vi "Fancy Dialog Box (LVOOP).vi"() -> ()   [LabVIEW 2012]
doc: "This example shows how to use the UI Tools Dialog classes to create fancy dialog boxes with background blackening."
uses:
  _Commands_Example.ctl
  Dialog/Dialog/Dialog/Dialog.lvclass
  Dialog/ListSelection/Selection Mode.ctl
  Dialog/MessageBox/pictures/pictures.ctl
  Fading/_Fade In(I32).vi
  Fading/_Fade Out(I32).vi
  Dialog/MessageBox/MessageBox.lvclass
  Dialog/Msg_Error/Msg_Error.lvclass
  Dialog/ListSelection/ListSelection.lvclass
panel:
  in  "Error\nDialog":bool caption="Press this button to simulate a dialog box call."
  in  "Alarm\nDialog":bool caption="Press this button to simulate a dialog box call."
  in  "Selection\nList":bool caption="Press this button to simulate a dialog box call."
  in  "One-button\nDialog":bool caption="Press this button to simulate a dialog box call."
  in  "Exit":bool caption="Exits with a fade out"
  # "Press the ? button to call up a Dialog Box using classes.\nPress Exit to Fade out and quit."
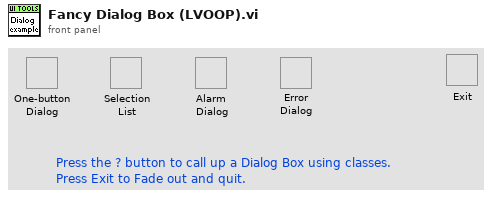
[diagram p1: front panel]
types:
  T1 = typedef "_Commands_Example.ctl" = enum16{"Idle", "Init", "OpenFP", "CloseFP", "Fade - Partial", "About", "Exit"}
  T2 = typedef "ListSelection.lvlib/ListSelection.lvclass/Selection Mode.ctl" = enum16{"Zero or one", "One", "Zero or more", "One or more"}
  T3 = typedef "pictures.ctl" = enum16{"Alarm", "Download", "Edition", "Encrypted", "Error", "Hardware Information", "Important", "Memory", "Network", "Package", "Password", "Readme", "Search", "System", "USB", "User", "Wireless", "www"}
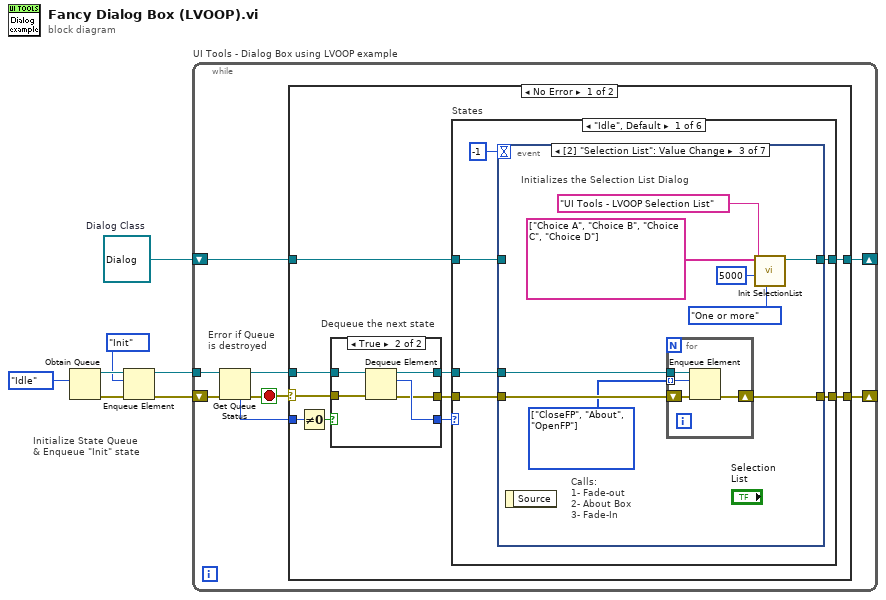
[diagram p0: block diagram]
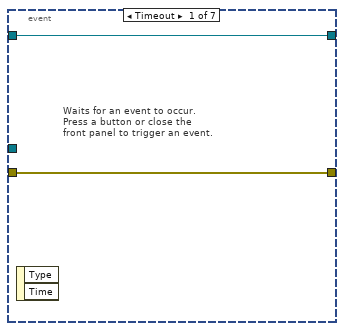
[diagram p2: hidden frame]
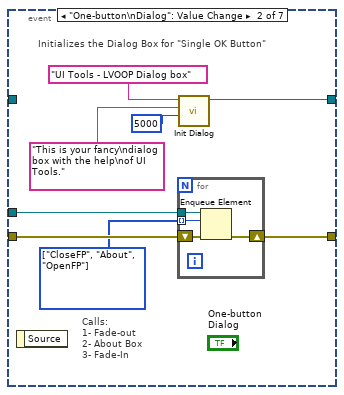
[diagram p3: hidden frame]
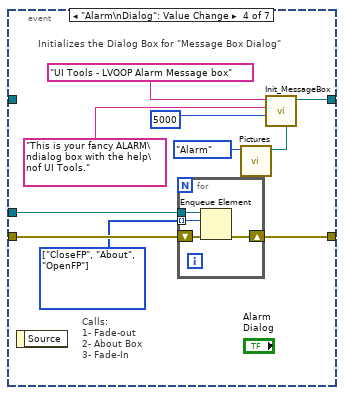
[diagram p4: hidden frame]
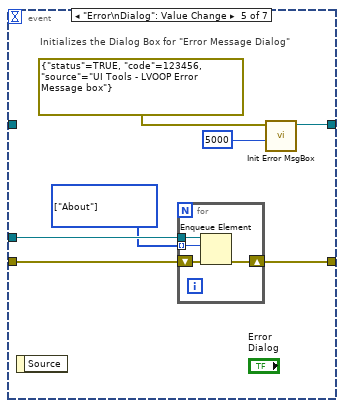
[diagram p5: hidden frame]
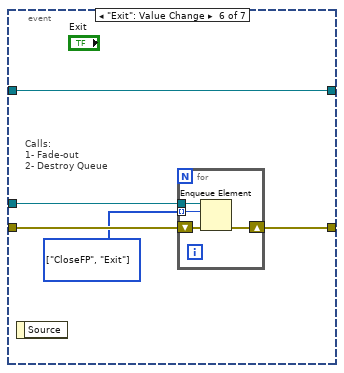
[diagram p6: hidden frame]
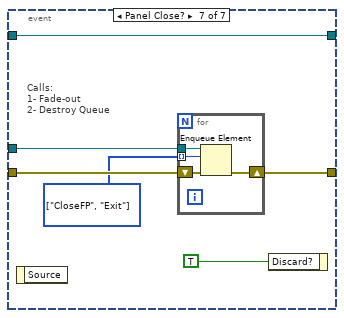
[diagram p7: hidden frame]
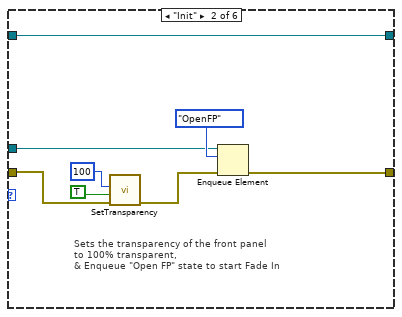
[diagram p8: hidden frame]
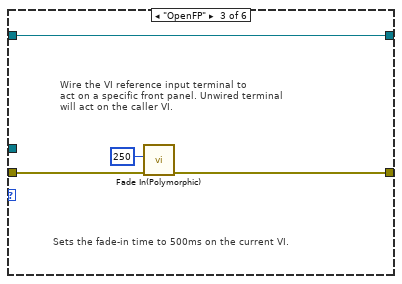
[diagram p9: hidden frame]
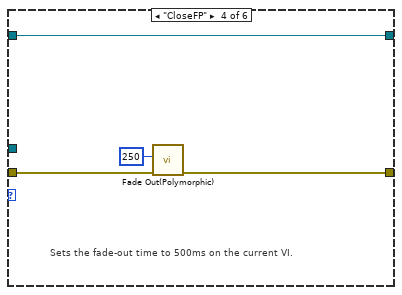
[diagram p10: hidden frame]
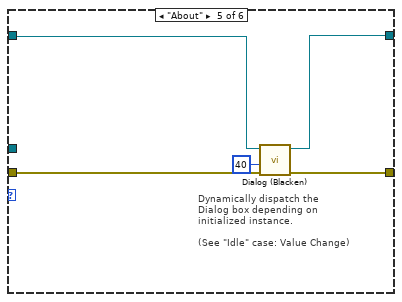
[diagram p11: hidden frame]
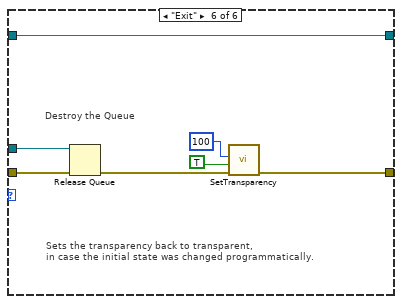
[diagram p12: hidden frame]
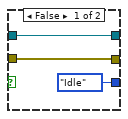
[diagram p13: hidden frame]
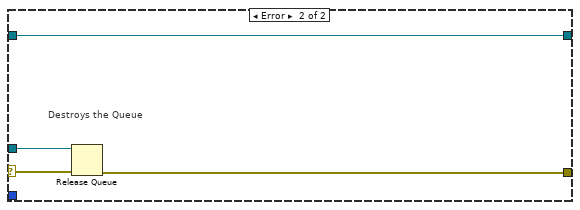
[diagram p14: hidden frame]
diagram:
  w1 = refnum<class "Dialog.lvclass"> refnum  # Dialog Class
  # "Initialize State Queue\n& Enqueue \"Init\" state"
  n1 = Obtain Queue(element data type=_Commands_Example."Idle" ("Commands")) -> (queue out=w7:refnum<queue>, error out=w5:errorcluster)  [unwired: 3 in, 2 out]
  n2 = Enqueue Element(queue=w7, element=_Commands_Example."Init" ("Commands"), error in (no error)=w5) -> (queue out=w3:refnum<queue>, error out=w4:errorcluster)  [unwired: 2 out]
  n3 = while "UI Tools - Dialog Box using LVOOP example" {
    tunnel: w3 -> [w14]
    shift-right: [w10] -> _
    shift-left: w4 -> [w15]
    shift-right: [w8] -> _
    shift-left: w1 -> [w9]
    stop <- w12 stop-if-true
    # "Error if Queue\nis destroyed"
    n4 = Get Queue Status(queue=w14, error in (no error)=w15) -> (queue out=w11:refnum<queue>, error out=w12:errorcluster, # elements in queue=w13:i32)  [unwired: 6 out]
    n5 = case shown="No Error" w12 {
      selector: w12 -> [w22 w141]
      tunnel: w13 -> [w25 _]
      tunnel: w11 -> [w23 w142]
      tunnel: [w18 w140] -> w10
      tunnel: w9 -> [w17 w139]
      tunnel: [w16 w139] -> w8
      frame No Error {
        # "Dequeue the next state"
        n6 = Not Equal To 0?(x=w25) -> (x != 0?=w24:bool)
        n7 = case shown="True" w24 {
          tunnel: w23 -> [w133 w138]
          tunnel: w22 -> [w132 w137]
          tunnel: [_Commands_Example."Idle" ("Commands") w136] -> w21
          tunnel: [w133 w135] -> w20
          tunnel: [w132 w134] -> w19
          frame False {
          }
          frame True {
            n8 = Dequeue Element(queue=w138, error in (no error)=w137) -> (queue out=w135:refnum<queue>, element=w136:T1, error out=w134:errorcluster)  [unwired: 2 out]
          }
        }
        n9 = case "States" shown="\"Idle\", Default" w21 {
          tunnel: w20 -> [w30 w109 _ _ _ w129]
          tunnel: w19 -> [w29 w105 w113 w117 w120 w130]
          tunnel: [w28 w104 w112 w116 w123 w125] -> w18
          tunnel: w17 -> [w27 w103 w111 w115 w122 w124]
          tunnel: [w26 w103 w111 w115 w121 w124] -> w16
          frame "Idle", Default {
            n10 = event shown="[2] \"Selection List\": Value Change" {
              selector: _ -> [_ _ _ _ _ _ _]
              dyn-events: _ -> [_ _ _ _ _ _ _]
              timeout: -1 -> [_ _ _ _ _ _ _]
              tunnel: w30 -> [_ w41 w54 w68 w79 w88 w98]
              tunnel: w29 -> [w33 w40 w53 w67 w78 w87 w97]
              tunnel: [w33 w38 w51 w65 w77 w85 w95] -> w28
              tunnel: w27 -> [w32 _ _ _ _ w84 w93]
              tunnel: [w32 w37 w48 w64 w76 w84 w93] -> w26
              event Timeout {
                # "Waits for an event to occur.\nPress a button or close the\nfront panel to trigger an event."
                n11 = event-data() -> ()  [unwired: 3 out]
              }
              event "One-button\nDialog": Value Change {
                w39 = T1[] [enum."CloseFP", enum."About", enum."OpenFP"] items=["Idle", "Init", "OpenFP", "CloseFP", "Fade - Partial", "About", "Exit"]
                # "Initializes the Dialog Box for \"Single OK Button\""
                # "Calls: \n1- Fade-out\n2- About Box\n3- Fade-In"
                n12 = event-data() -> ()  [unwired: 2 out]
                n13 = for {
                  tunnel: w41 -> [w45]
                  tunnel: w39 -> [w43] mode=indexing
                  shift-right: [w42] -> w38
                  shift-left: w40 -> [w44]
                  n14 = Enqueue Element(queue=w45, element=w43, error in (no error)=w44) -> (error out=w42:errorcluster)  [unwired: 3 out]
                }
                n15 = call "Init Dialog.vi"("Timeout (-1)"=5000, "Message"="This is your fancy\ndialog box with the help\nof UI Tools.", "Dialog Title"="UI Tools - LVOOP Dialog box" ("message")) -> ("Dialog out"=w37:refnum<class "Dialog.lvclass">)  [unwired: 3 in, 5 out]
              }
              event "Selection\nList": Value Change {
                w52 = T1[] [enum."CloseFP", enum."About", enum."OpenFP"] items=["Idle", "Init", "OpenFP", "CloseFP", "Fade - Partial", "About", "Exit"]
                # "Initializes the Selection List Dialog"
                # "Calls: \n1- Fade-out\n2- About Box\n3- Fade-In"
                n16 = event-data() -> ()  [unwired: 2 out]
                n17 = for {
                  tunnel: w54 -> [w58]
                  tunnel: w52 -> [w56] mode=indexing
                  shift-right: [w55] -> w51
                  shift-left: w53 -> [w57]
                  n18 = Enqueue Element(queue=w58, element=w56, error in (no error)=w57) -> (error out=w55:errorcluster)  [unwired: 3 out]
                }
                n19 = call "Init SelectionList.vi"("Selection Mode"=Selection_Mode."One or more", "Timeout (-1)"=5000, "Items List"=string[] ["Choice A", "Choice B", "Choice C", "Choice D"], "Message"="UI Tools - LVOOP Selection List" ("message")) -> ("ListSelection out"=w48:refnum<class "ListSelection.lvclass">)  [unwired: 6 in, 1 out]
              }
              event "Alarm\nDialog": Value Change {
                w66 = T1[] [enum."CloseFP", enum."About", enum."OpenFP"] items=["Idle", "Init", "OpenFP", "CloseFP", "Fade - Partial", "About", "Exit"]
                # "Initializes the Dialog Box for \"Message Box Dialog\""
                # "Calls: \n1- Fade-out\n2- About Box\n3- Fade-In"
                n20 = event-data() -> ()  [unwired: 2 out]
                n21 = for {
                  tunnel: w68 -> [w72]
                  tunnel: w66 -> [w70] mode=indexing
                  shift-right: [w69] -> w65
                  shift-left: w67 -> [w71]
                  n22 = Enqueue Element(queue=w72, element=w70, error in (no error)=w71) -> (error out=w69:errorcluster)  [unwired: 3 out]
                }
                n23 = call "Pictures.vi"("Pictures"=pictures."Alarm") -> ("Path"=w60:path)  [unwired: 10 out]
                n24 = call "Init_MessageBox.vi"("Image path"=w60, "Timeout (-1)"=5000, "Message"="This is your fancy ALARM\ndialog box with the help\nof UI Tools.", "MsgBox Title"="UI Tools - LVOOP Alarm Message box" ("message")) -> ("MessageBox out"=w64:refnum<class "MessageBox.lvclass">)  [unwired: 3 in, 4 out]
              }
              event "Error\nDialog": Value Change {
                w73 = T1[] [enum."About"] items=["Idle", "Init", "OpenFP", "CloseFP", "Fade - Partial", "About", "Exit"]
                # "Initializes the Dialog Box for \"Error Message Dialog\""
                n25 = event-data() -> ()  [unwired: 2 out]
                n26 = for {
                  tunnel: w79 -> [w83]
                  tunnel: w73 -> [w81] mode=indexing
                  shift-right: [w80] -> w77
                  shift-left: w78 -> [w82]
                  n27 = Enqueue Element(queue=w83, element=w81, error in (no error)=w82) -> (error out=w80:errorcluster)  [unwired: 3 out]
                }
                n28 = call "Init Error MsgBox.vi"("Timeout (-1)"=5000, "Error"=errorcluster {"status"=TRUE, "code"=123456, "source"="UI Tools - LVOOP Error Message box"} ("error out")) -> ("Msg_Error out"=w76:refnum<class "Msg_Error.lvclass">)  [unwired: 5 in, 4 out]
              }
              event "Exit": Value Change {
                w86 = T1[] [enum."CloseFP", enum."Exit"] items=["Idle", "Init", "OpenFP", "CloseFP", "Fade - Partial", "About", "Exit"]
                # "Calls: \n1- Fade-out\n2- Destroy Queue"
                n29 = event-data() -> ()  [unwired: 2 out]
                n30 = for {
                  tunnel: w88 -> [w92]
                  tunnel: w86 -> [w90] mode=indexing
                  shift-right: [w89] -> w85
                  shift-left: w87 -> [w91]
                  n31 = Enqueue Element(queue=w92, element=w90, error in (no error)=w91) -> (error out=w89:errorcluster)  [unwired: 3 out]
                }
              }
              event Panel Close? {
                w96 = T1[] [enum."CloseFP", enum."Exit"] items=["Idle", "Init", "OpenFP", "CloseFP", "Fade - Partial", "About", "Exit"]
                # "Calls: \n1- Fade-out\n2- Destroy Queue"
                n32 = event-data() -> ()  [unwired: 2 out]
                n33 = for {
                  tunnel: w98 -> [w102]
                  tunnel: w96 -> [w100] mode=indexing
                  shift-right: [w99] -> w95
                  shift-left: w97 -> [w101]
                  n34 = Enqueue Element(queue=w102, element=w100, error in (no error)=w101) -> (error out=w99:errorcluster)  [unwired: 3 out]
                }
                n35 = event-data("Discard?"=TRUE) -> ()  [unwired: 1 in, 1 out]
              }
            }
          }
          frame "Init" {
            # "Sets the transparency of the front panel\nto 100% transparent,\n& Enqueue \"Open FP\" state to start Fade In"
            n36 = call "SetTransparency.vi"("error in"=w105, "Run VI Transparently (T)"=TRUE, "Transparency (%)"=100) -> ("error out"=w106:errorcluster)  [unwired: 1 in, 7 out]
            n37 = Enqueue Element(queue=w109, element=_Commands_Example."OpenFP" ("Commands"), error in (no error)=w106) -> (error out=w104:errorcluster)  [unwired: 3 out]
          }
          frame "OpenFP" {
            # "Wire the VI reference input terminal to\nact on a specific front panel. Unwired terminal\nwill act on the caller VI."
            # "Sets the fade-in time to 500ms on the current VI."
            n38 = call-poly "Fade In(Polymorphic).vi"("error in"=w113, "Fade time (ms)"=250) -> ("error out"=w112:errorcluster)  [unwired: 2 in, 7 out]
          }
          frame "CloseFP" {
            # "Sets the fade-out time to 500ms on the current VI."
            n39 = call-poly "Fade Out(Polymorphic).vi"("error in"=w117, "Fade time (ms)"=250) -> ("error out"=w116:errorcluster)  [unwired: 2 in, 7 out]
          }
          frame "About" {
            # "Dynamically dispatch the\nDialog box depending on \ninitialized instance.\n\n(See \"Idle\" case: Value Change)"
            n40 = call-dynamic "Dialog (Blacken).vi"("error in (no error)"=w120, "Transparency (40)"=u8 40, "Dialog in"=w122) -> ("error out"=w123:errorcluster, "Dialog out"=w121:refnum<class "Dialog.lvclass">)  [unwired: 7 out]
          }
          frame "Exit" {
            # "Destroy the Queue"
            # "Sets the transparency back to transparent, \nin case the initial state was changed programmatically."
            n41 = Release Queue(queue=w129, error in (no error)=w130) -> (error out=w126:errorcluster)  [unwired: 3 out]
            n42 = call "SetTransparency.vi"("error in"=w126, "Run VI Transparently (T)"=TRUE, "Transparency (%)"=100) -> ("error out"=w125:errorcluster)  [unwired: 1 in, 7 out]
          }
        }
      }
      frame Error {
        # "Destroys the Queue"
        n43 = Release Queue(queue=w142, error in (no error)=w141) -> (error out=w140:errorcluster)  [unwired: 3 out]
      }
    }
  }
